vi "VALCCS_main_vi_ver_1.5.vi"() -> ()   [LabVIEW 2019]
uses:
  <vilib>/Utility/NIReport.llb/Report Type.ctl
  <vilib>/Utility/NIReport.llb/Append Report Text (str wrap).vi
  <vilib>/Utility/NIReport.llb/NI_report.lvclass
  <vilib>/Utility/NIReport.llb/NI_ReportGenerationCore.lvlib
panel:
  in  "Tab Control":enum32{"Report Generation", "CG Calculation"}(tab)
  in  "Report Title":string="20"
  in  "Test Performer Name":string="70"
  in  "Customer Name":string="100"
  in  "Reicieve Date":string
  out "Total Weight (KG)":dbl(graph)
  out "Load Cell 1 Weight (KG)":dbl(graph)
  out "Load Cell 2 Weight (KG)":dbl(graph)
  out "Voltage 1":dbl
  out "Weight 1":dbl
  out "Rounded weight 1":dbl
  in  "Log Axle 1 Load (KG)":bool
  in  "Log Axle 2 Load (KG)":bool
  in  "Log Axle 3 Load (KG)":bool
  out "Axle 1 Load":dbl
  out "Axle 3 Load":dbl
  out "Axle 2 Load":dbl
  in  "Axle 1 to 3 distance (mm)":dbl
  in  "Axle 2 to 3 distance (mm)":dbl
  out "CG from Axle 1 (mm)":dbl
  in  "stop (F)":bool
  out "Total Weight (KG)":dbl
  out "Voltage 2":dbl
  out "Weight 2":dbl
  out "Rounded weight 2":dbl
  # "Please Enter the Following Details for Automatic Report Generation."
  # "Date of Reception of UUT."
  # "Title of the Test Report."
  # "Name of the Customer."
  # "Name of the Test Performer."
  # "1"
  # "2"
  # "3"
  # "COG Calculation via Axle Load Measurement"
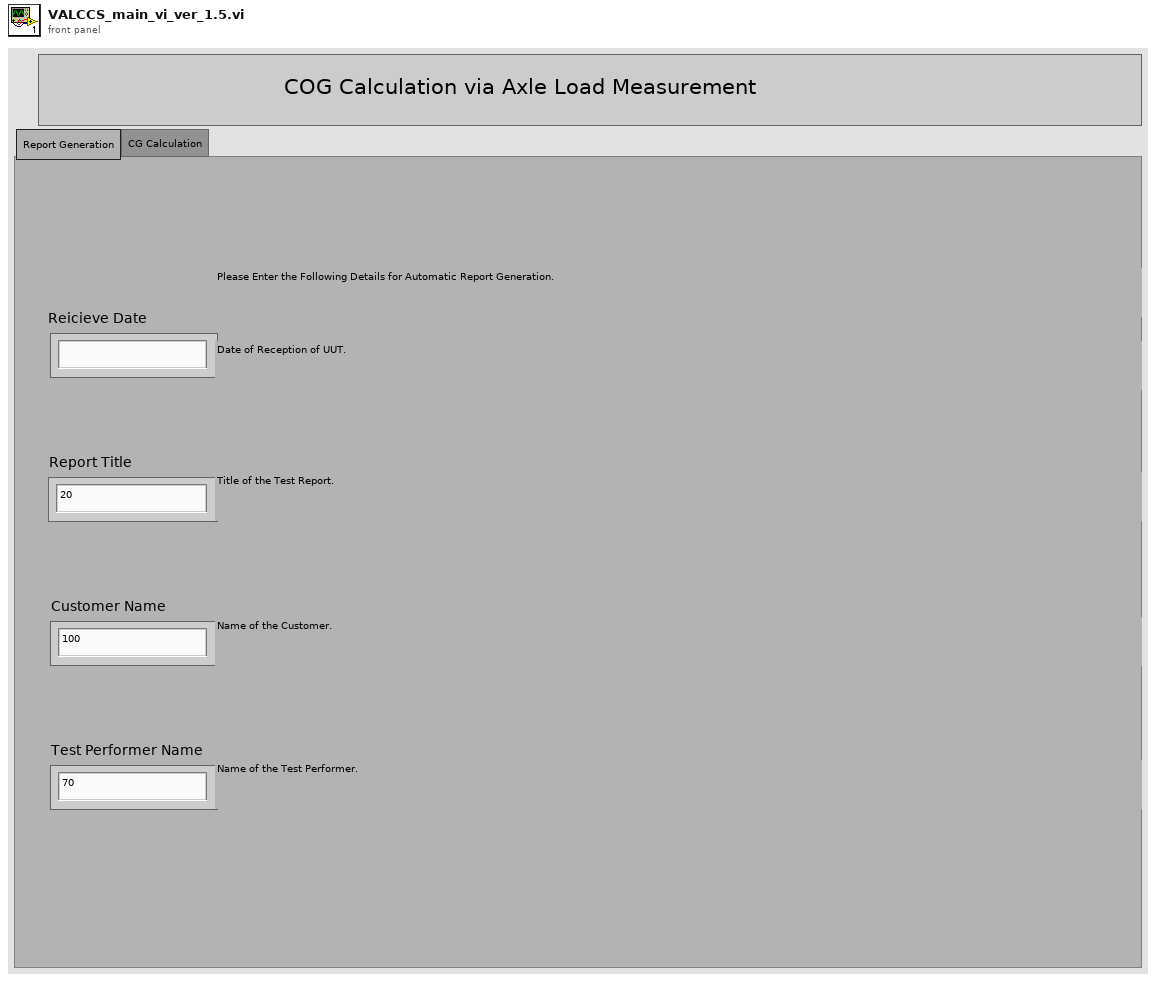
[diagram p1: front panel]
types:
  T1 = cluster{"position (Excel)":cluster{"row":i32, "column":i32}, "name (Excel)":string, "bookmark (Word)":string}
  T2 = typedef "NI_ReportGenerationCore.lvlib/Report Type.ctl" = enum16{"HTML", "Word", "Excel"}
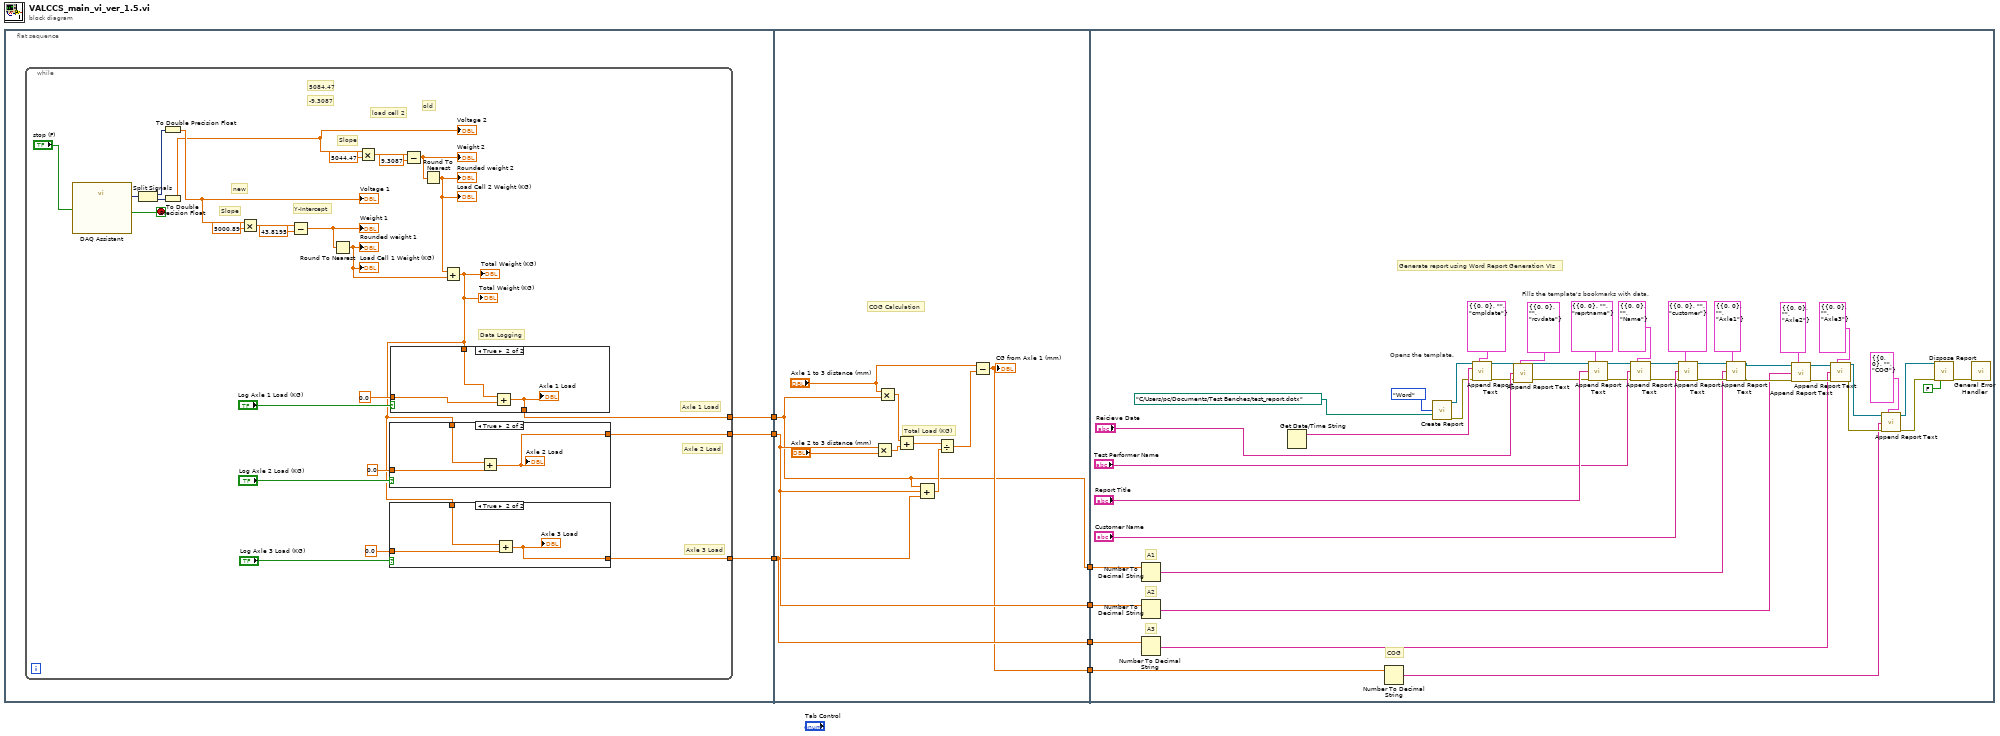
[diagram p0: block diagram]
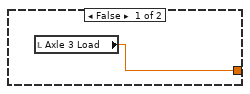
[diagram p2: hidden frame]
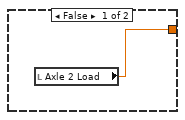
[diagram p3: hidden frame]
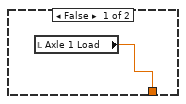
[diagram p4: hidden frame]
diagram:
  n1 = flat-sequence {
    tunnel: [w10] -> w7
    tunnel: [w9] -> w6
    tunnel: [w8] -> w5
    tunnel: w7 -> [w55]
    tunnel: w6 -> [w51]
    tunnel: w5 -> [w56]
    tunnel: [w51] -> w4
    tunnel: [w56] -> w3
    tunnel: [w55] -> w2
    tunnel: [w54] -> w1
    tunnel: w4 -> [w68]
    tunnel: w3 -> [w66]
    tunnel: w2 -> [w64]
    tunnel: w1 -> [w62]
    frame #0 {
      n2 = while {
        tunnel: [w30] -> w9
        tunnel: [w29] -> w8
        tunnel: [w28] -> w10
        stop <- w14 stop-if-true
        # "new"
        # "old"
        # "-9.3087"
        # "5084.47"
        # "Slope"
        # "load cell 2"
        # "Axle 3 Load"
        # "Axle 1 Load"
        # "Axle 2 Load"
        # "Data Logging"
        # "Slope"
        # "Y-Intercept"
        n3 = call "DAQ Assistant"("stop (F)"="stop (F)") -> ("data"=w15:dynamicdata, "stopped"=w14:bool)  [unwired: 15 in, 2 out]
        n4 = Split Signals(w15) -> (w17:dynamicdata, w16:dynamicdata)  [unwired: 2 in]
        n5 = To Double Precision Float(number=w17) -> (double precision float=w12:dbl)
        "Voltage 1" <- w12
        n6 = To Double Precision Float(number=w16) -> (double precision float=w11:dbl)
        "Voltage 2" <- w11
        n7 = Multiply(x=w12, y=5000.89) -> (x*y=w26:dbl)
        n8 = Subtract(x=w26, y=43.8195) -> (x-y=w25:dbl)
        "Weight 1" <- w25
        n9 = Round To Nearest(number=w25) -> (nearest integer value=w24:dbl)
        "Load Cell 1 Weight (KG)" <- w24
        "Rounded weight 1" <- w24
        n10 = Multiply(x=w11, y=5044.47) -> (x*y=w20:dbl)
        n11 = Subtract(x=w20, y=9.3087) -> (x-y=w19:dbl)
        "Weight 2" <- w19
        n12 = Round To Nearest(number=w19) -> (nearest integer value=w18:dbl)
        "Load Cell 2 Weight (KG)" <- w18
        "Rounded weight 2" <- w18
        n13 = Add(x=w18, y=w24) -> (x+y=w23:dbl)
        "Total Weight (KG)" <- w23
        "Total Weight (KG)" <- w23
        n14 = case shown="True" "Log Axle 2 Load (KG)" {
          tunnel: w23 -> [_ w45]
          tunnel: 0.0 -> [_ w44]
          tunnel: [w42 w43] -> w29
          frame False {
            n15 = local read "Axle 2 Load"() -> (w42:dbl)
          }
          frame True {
            n16 = Add(x=w45, y=w44) -> (x+y=w43:dbl)
            "Axle 2 Load" <- w43
          }
        }
        n17 = case shown="True" "Log Axle 3 Load (KG)" {
          tunnel: w23 -> [_ w40]
          tunnel: 0.0 -> [_ w41]
          tunnel: [w38 w39] -> w28
          frame False {
            n18 = local read "Axle 3 Load"() -> (w38:dbl)
          }
          frame True {
            n19 = Add(x=w40, y=w41) -> (x+y=w39:dbl)
            "Axle 3 Load" <- w39
          }
        }
        n20 = case shown="True" "Log Axle 1 Load (KG)" {
          tunnel: 0.0 -> [_ w48]
          tunnel: w23 -> [_ w49]
          tunnel: [w46 w47] -> w30
          frame False {
            n21 = local read "Axle 1 Load"() -> (w46:dbl)
          }
          frame True {
            n22 = Add(x=w49, y=w48) -> (x+y=w47:dbl)
            "Axle 1 Load" <- w47
          }
        }
      }
    }
    frame #1 {
      # "COG Calculation"
      # "Total Load (KG)"
      n23 = Multiply(x=w56, y="Axle 2 to 3 distance (mm)") -> (x*y=w52:dbl)
      n24 = Multiply(x="Axle 1 to 3 distance (mm)", y=w51) -> (x*y=w53:dbl)
      n25 = Add(x=w53, y=w52) -> (x+y=w58:dbl)
      n26 = Compound Arithmetic op=ADD(w51, w56, w55) -> (w59:dbl)
      n27 = Divide(x=w58, y=w59) -> (x/y=w60:dbl)
      n28 = Subtract(x="Axle 1 to 3 distance (mm)", y=w60) -> (x-y=w54:dbl)
      "CG from Axle 1 (mm)" <- w54
    }
    frame #2 {
      # "COG"
      # "A3"
      # "A2"
      # "A1"
      # "Generate report using Word Report Generation VIs"
      # "Fills the template's bookmarks with data."
      # "Opens the template."
      n29 = Number To Decimal String(number=w68) -> (decimal integer string=w67:string)  [unwired: 1 in]
      n30 = Number To Decimal String(number=w66) -> (decimal integer string=w65:string)  [unwired: 1 in]
      n31 = Number To Decimal String(number=w64) -> (decimal integer string=w63:string)  [unwired: 1 in]
      n32 = Get Date/Time String() -> (date string=w106:string)  [unwired: 3 in, 1 out]
      n33 = Number To Decimal String(number=w62) -> (decimal integer string=w61:string)  [unwired: 1 in]
      n34 = call <vilib>:"Create Report.vi"("report type"=Report_Type."Word", "template (empty)"=path "C:/Users/pc/Documents/Test Benches/test_report.dotx") -> ("report out"=w87:refnum<class "NI_report.lvclass">, "error out"=w86:errorcluster)  [unwired: 12 in]
      n35 = call-poly <vilib>:"Append Report Text.vi"("report in"=w87, "MS Office parameters"=T1 {"position (Excel)"={"row"=0, "column"=0}, "name (Excel)"="", "bookmark (Word)"="cmpldate"}, "text"=w106, "error in (no error)"=w86) -> ("report out"=w83:refnum<class "NI_report.lvclass">, "error out"=w82:errorcluster)  [unwired: 8 in, 2 out]
      n36 = call-poly <vilib>:"Append Report Text.vi"("report in"=w83, "MS Office parameters"=T1 {"position (Excel)"={"row"=0, "column"=0}, "name (Excel)"="", "bookmark (Word)"="rcvdate"}, "text"="Reicieve Date", "error in (no error)"=w82) -> ("report out"=w81:refnum<class "NI_report.lvclass">, "error out"=w80:errorcluster)  [unwired: 8 in, 2 out]
      n37 = call-poly <vilib>:"Append Report Text.vi"("report in"=w81, "MS Office parameters"=T1 {"position (Excel)"={"row"=0, "column"=0}, "name (Excel)"="", "bookmark (Word)"="reprtname"}, "text"="Report Title", "error in (no error)"=w80) -> ("report out"=w96:refnum<class "NI_report.lvclass">, "error out"=w99:errorcluster)  [unwired: 8 in, 2 out]
      n38 = call-poly <vilib>:"Append Report Text.vi"("report in"=w96, "MS Office parameters"=T1 {"position (Excel)"={"row"=0, "column"=0}, "name (Excel)"="", "bookmark (Word)"="Name"}, "text"="Test Performer Name", "error in (no error)"=w99) -> ("report out"=w95:refnum<class "NI_report.lvclass">, "error out"=w98:errorcluster)  [unwired: 8 in, 2 out]
      n39 = call-poly <vilib>:"Append Report Text.vi"("report in"=w95, "MS Office parameters"=T1 {"position (Excel)"={"row"=0, "column"=0}, "name (Excel)"="", "bookmark (Word)"="customer"}, "text"="Customer Name", "error in (no error)"=w98) -> ("report out"=w94:refnum<class "NI_report.lvclass">, "error out"=w97:errorcluster)  [unwired: 8 in, 2 out]
      n40 = call-poly <vilib>:"Append Report Text.vi"("report in"=w94, "MS Office parameters"=T1 {"position (Excel)"={"row"=0, "column"=0}, "name (Excel)"="", "bookmark (Word)"="Axle1"}, "text"=w67, "error in (no error)"=w97) -> ("report out"=w77:refnum<class "NI_report.lvclass">, "error out"=w76:errorcluster)  [unwired: 8 in, 2 out]
      n41 = call-poly <vilib>:"Append Report Text.vi"("report in"=w77, "MS Office parameters"=T1 {"position (Excel)"={"row"=0, "column"=0}, "name (Excel)"="", "bookmark (Word)"="Axle2"}, "text"=w65, "error in (no error)"=w76) -> ("report out"=w75:refnum<class "NI_report.lvclass">, "error out"=w74:errorcluster)  [unwired: 8 in, 2 out]
      n42 = call-poly <vilib>:"Append Report Text.vi"("report in"=w75, "MS Office parameters"=T1 {"position (Excel)"={"row"=0, "column"=0}, "name (Excel)"="", "bookmark (Word)"="Axle3"}, "text"=w63, "error in (no error)"=w74) -> ("report out"=w72:refnum<class "NI_report.lvclass">, "error out"=w71:errorcluster)  [unwired: 8 in, 2 out]
      n43 = call-poly <vilib>:"Append Report Text.vi"("report in"=w72, "MS Office parameters"=T1 {"position (Excel)"={"row"=0, "column"=0}, "name (Excel)"="", "bookmark (Word)"="COG"}, "text"=w61, "error in (no error)"=w71) -> ("report out"=w70:refnum<class "NI_report.lvclass">, "error out"=w69:errorcluster)  [unwired: 8 in, 2 out]
      n44 = call-dynamic "Dispose Report.vi"("report in"=w70, "error in (no error)"=w69, "close report? (T)"=FALSE ("Close Report? (T)")) -> ("error out"=w102:errorcluster)  [unwired: 12 in]
      n45 = call <vilib>:"General Error Handler.vi"("error in (no error)"=w102) -> ()  [unwired: 10 in, 5 out]
    }
  }
